vi "SAC-Write Text File.vi"(0 "Params":T1, 5 "State":T5, 7 "Data":dbl[](array[numeric]), 9 "Stimulus":dbl[](array[numeric]), 11 "error in (no error)":errorcluster, 12 "Actual Fs":dbl) -> (15 "error out":errorcluster)   [LabVIEW 2020]
uses:
  Typedefs/SAC-State.ctl
  Typedefs/SAC-Parameters.ctl
  HRTF VIs/Typedefs/HRTF-Waveform.ctl
  HRTF VIs/Typedefs/HRTF-Window.ctl
  HRTF VIs/Typedefs/HRTF-Window Type.ctl
panel:
  in  "Result":cluster{"Stimulus":dbl[], "Response":dbl[]}
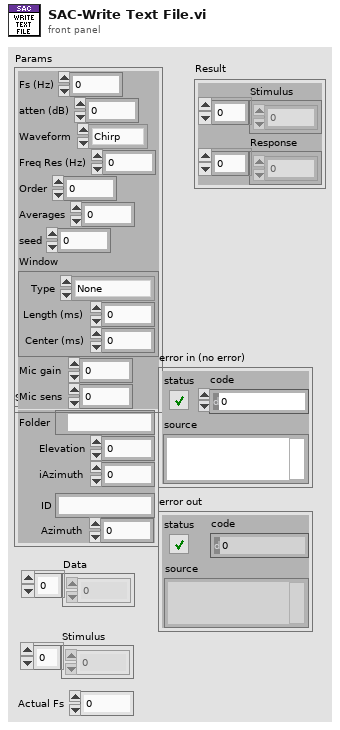
[diagram p1: front panel]
types:
  T1 = typedef "SAC-Parameters.ctl" = cluster{"Fs (Hz)":dbl, "atten (dB)":dbl, "Waveform":T2, "Freq Res (Hz)":dbl, "Order":i32, "Averages":i32, "seed":i64, "Window":T3, "Mic gain":dbl, "Mic sens":dbl}
  T2 = typedef "HRTF-Waveform.ctl" = enum16{"Chirp", "MLS"}
  T3 = typedef "HRTF-Window.ctl" = cluster{"Type":T4, "Length (ms)":dbl, "Center (ms)":dbl}
  T4 = typedef "HRTF-Window Type.ctl" = enum16{"None", "Rectangle", "Hanning"}
  T5 = typedef "SAC-State.ctl" = cluster{"Folder":path, "Elevation":dbl, "iAzimuth":i32, "ID":string, "Azimuth":dbl}
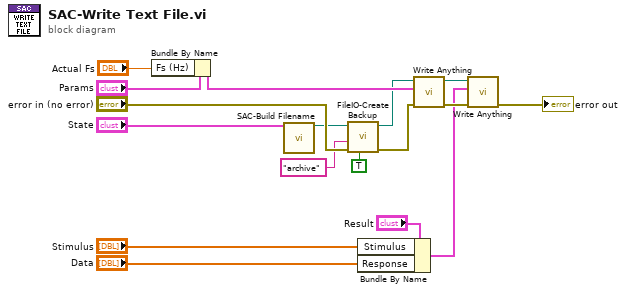
[diagram p0: block diagram]
diagram:
  n1 = Bundle By Name(cluster="Params", "Fs (Hz)"="Actual Fs") -> (w6:T1)
  n2 = call "SAC-Build Filename.vi"("State"="State") -> ("path"=w5:path)  [unwired: 13 in, 1 out]
  n3 = call "FileIO-Create Backup.vi"("Append date"=TRUE, "error in (no error)"="error in (no error)", "Subfolder"="archive", "Path"=w5) -> ("error out"=w3:errorcluster, "Path (thru)"=w2:path)  [unwired: 4 in, 2 out]
  n4 = Bundle By Name(cluster="Result", "Stimulus"="Stimulus", "Response"="Data") -> (w7:cluster{"Stimulus":dbl[], "Response":dbl[]})
  n5 = call "Write Anything.vi"("Error In"=w3, "Anything"=w6, "Path (dialog)"=w2) -> ("Error Out"=w10:errorcluster, "Path out"=w9:path)  [unwired: 7 in]
  n6 = call "Write Anything.vi"("Error In"=w10, "Anything"=w7, "Path (dialog)"=w9) -> ("Error Out"=→"error out":errorcluster)  [unwired: 7 in, 1 out]
